vi "Trim Sensitivity Characterization.vi"(0 "TSM context":T1, 5 "Start":dbl=1.0, 7 "Delta":dbl format="%#_13g", 9 "End":dbl=1.0) -> (4 "Sens Target":dbl[](array[numeric]), 6 "Trimmed dB V":dbl[][](array[numeric]), 15 "error out":errorcluster)   [LabVIEW 2020]
uses:
  <vilib>/NI_TestStand_SemiconductorModule/NI_TestStand_Semiconductor_Module.lvlibp/PinMap/General/SemiconductorModuleContext.ctl
  <vilib>/NI_TestStand_SemiconductorModule/NI_TestStand_Semiconductor_Module.lvlibp
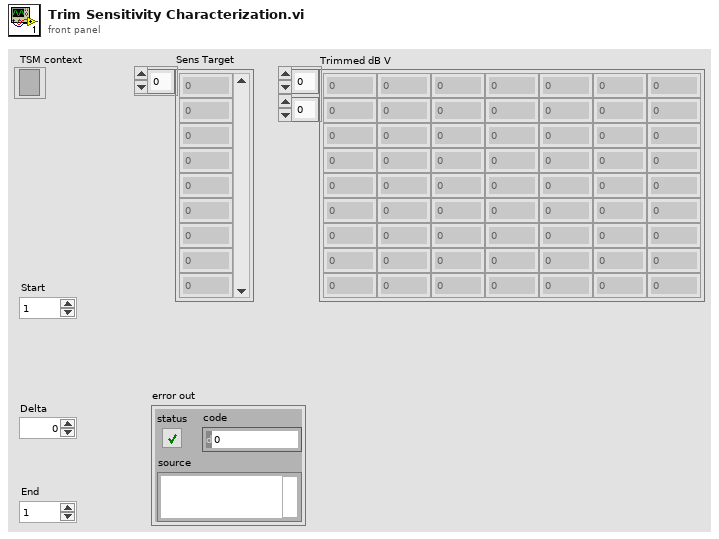
[diagram p1: front panel]
types:
  T1 = typedef "NI_TestStand_Semiconductor_Module.lvlibp/SemiconductorModuleContext.ctl" = refnum<k7>
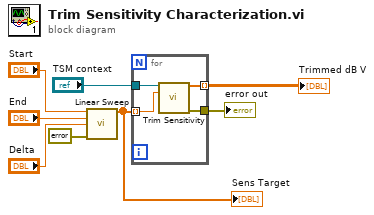
[diagram p0: block diagram]
diagram:
  n1 = call "Linear Sweep.vi"("Start"="Start", "End"="End", "Delta"="Delta", "error in (no error)"=errorcluster {"status"=FALSE, "code"=0, "source"=""}) -> ("Ramp Pattern"=w5:dbl[])  [unwired: 10 in, 1 out]
  "Sens Target" <- w5
  n2 = for {
    tunnel: [w12] -> w7
    tunnel: "TSM context" -> [w11]
    tunnel: w5 -> [w10] mode=indexing
    tunnel: [w9] -> w1 mode=indexing
    n3 = call "Trim Sensitivity.vi"("TSM context"=w11, "Target Sensitivity (dBV)"=w10) -> ("Trimmed dB V"=w9:dbl[], "error out"=w12:errorcluster)  [unwired: 12 in]
  }
  "error out" <- w7
  "Trimmed dB V" <- w1
